vi "Set IPS Switch Heater.vi"(8 "error in (no error)":errorcluster, 10 "Switch Heater Status":T1, 11 "Instrument.Oxford1820 in":refnum<class "Instrument.Oxford1820.lvclass">) -> (0 "error out":errorcluster, 2 "Response":string, 3 "Instrument.Oxford1820 out":refnum<class "Instrument.Oxford1820.lvclass">)   [LabVIEW 2019, in "Instrument.Oxford1820.lvclass"]
uses:
  Instrument.Oxford1820.lvclass
  <instrlib>/Mercury iXX/Mercury iXX.lvlib
  <instrlib>/Mercury iXX/Public/Libraries/Magnet/Open/Open Magnet Device.vi
  <instrlib>/Mercury iXX/Public/Libraries/Magnet.lvlib
  <instrlib>/Mercury iXX/Public/Libraries/Magnet/Signals/Read/Persistant Current (Read).vi
  <instrlib>/Mercury iXX/Public/Libraries/Magnet/Signals/Read/Current (Read).vi
  <instrlib>/Mercury iXX/Public/Libraries/Magnet/Signals/Set/Switch Heater Status (Set).vi
  <instrlib>/Mercury iXX/Public/Controls/Response String.ctl
  <instrlib>/Mercury iXX/Public/Libraries/Magnet/Controls/Switch Heater.ctl
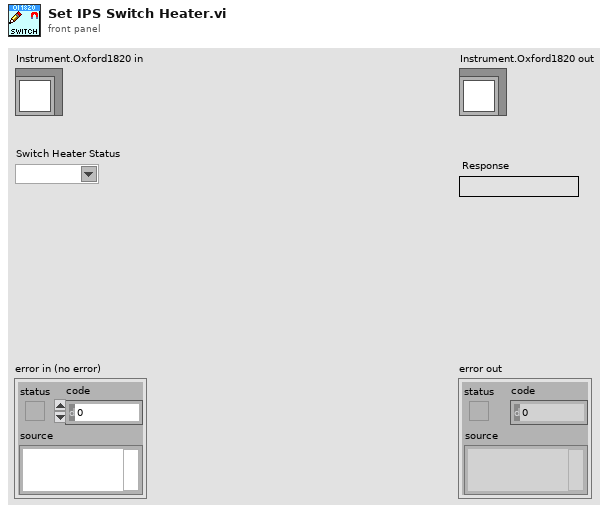
[diagram p1: front panel]
types:
  T1 = typedef "Mercury iXX.lvlib/Magnet.lvlib/Switch Heater.ctl" = string
  T2 = typedef "Mercury iXX.lvlib/Response String.ctl" = string
  T3 = typedef "Mercury iXX.lvlib/Mercury Reference.ctl" = cluster{"Comms":refnum<visa-resource-name>, "Device ID":string[], "Comms Layer":T4, "Command":string, "Query reference":T5}
  T4 = typedef "Mercury iXX.lvlib/Comms Transport Layer.ctl" = enum16{"Ethernet TCP/IP", "USB", "ISOBus - RS-232", "GPIB"}
  T5 = typedef "Mercury iXX.lvlib/Query Dynamic Reference.ctl" = refnum<vi>
  T6 = typedef "Mercury iXX.lvlib/Is Valid LED.ctl" = bool
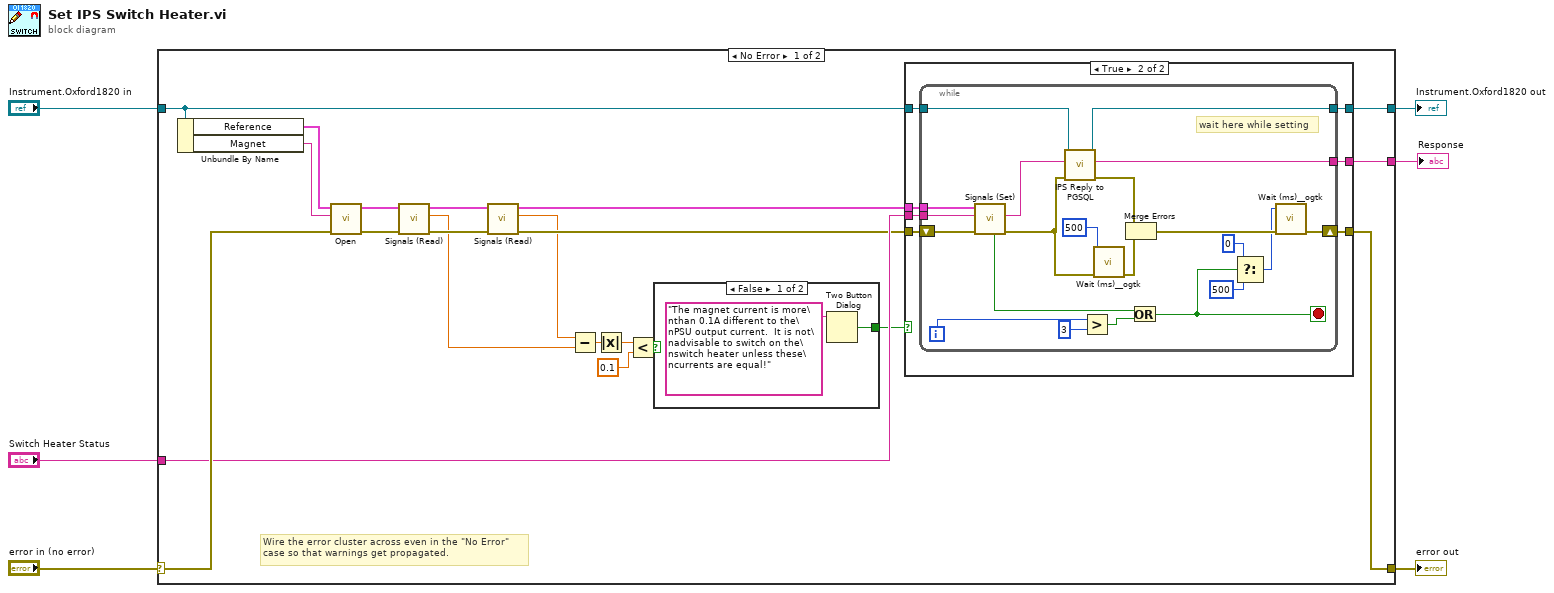
[diagram p0: block diagram]
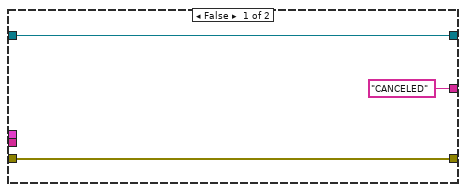
[diagram p2: hidden frame]
diagram:
  n1 = case shown="No Error" "error in (no error)" {
    selector: "error in (no error)" -> [w15 w62]
    tunnel: [w27 w62] -> w5
    tunnel: [w7 w61] -> w3
    tunnel: "Instrument.Oxford1820 in" -> [w8 w61]
    tunnel: [w26 _] -> w2
    tunnel: "Switch Heater Status" -> [w14 _]
    frame No Error {
      # "Wire the error cluster across even in the \"No Error\"\ncase so that warnings get propagated."
      n2 = Unbundle By Name(w8) -> ("Reference"=w25:T3, "Magnet"=w24:string)
      n3 = call-poly <instrlib>:"Open.vi"("error in (no error)"=w15, "Device Identifier"=w24, "Mercury Reference In"=w25) -> ("error out"=w18:errorcluster, "Mercury Reference Out"=w17:T3)  [unwired: 7 out]
      n4 = call-poly <instrlib>:"Signals (Read).vi"("error in"=w18, "Mercury Reference In"=w17) -> ("error out"=w20:errorcluster, "Current"=w10:dbl, "Mercury Reference Out"=w19:T3)  [unwired: 1 in, 6 out]
      n5 = call-poly <instrlib>:"Signals (Read).vi"("error in"=w20, "Mercury Reference In"=w19) -> ("error out"=w13:errorcluster, "Persistant Current"=w11:dbl, "Mercury Reference Out"=w12:T3)  [unwired: 1 in, 6 out]
      n6 = Subtract(x=w11, y=w10) -> (x-y=w21:dbl)
      n7 = Absolute Value(x=w21) -> (abs(x)=w22:dbl)
      n8 = Less?(x=w22, y=0.1) -> (x < y?=w23:bool)
      n9 = case shown="False" w23 {
        selector: w23 -> [_ w60]
        tunnel: [w59 w60] -> w9
        frame False {
          n10 = Two Button Dialog(message="The magnet current is more\nthan 0.1A different to the\nPSU output current.  It is not\nadvisable to switch on the\nswitch heater unless these\ncurrents are equal!") -> (T button?=w59:bool)  [unwired: 2 out]
        }
        frame True {
        }
      }
      n11 = case shown="True" w9 {
        tunnel: [w30 w37] -> w27
        tunnel: [T2 "CANCELED" ("Response") w36] -> w26
        tunnel: w8 -> [w28 w35]
        tunnel: w14 -> [_ w34]
        tunnel: w13 -> [w30 w33]
        tunnel: w12 -> [_ w32]
        tunnel: [w28 w31] -> w7
        frame False {
        }
        frame True {
          n12 = while {
            tunnel: [w46] -> w36
            tunnel: w35 -> [w48]
            tunnel: w34 -> [w55]
            tunnel: w32 -> [w56]
            shift-right: [w53] -> w37
            shift-left: w33 -> [w57]
            tunnel: [w47] -> w31
            i -> [w42]
            stop <- w40 stop-if-true
            # "wait here while setting"
            n13 = call-poly <instrlib>:"Signals (Set).vi"("error in"=w57, "Switch Heater Status"=w55, "Mercury Reference In"=w56) -> ("error out"=w51:errorcluster, "Response"=w46:T2, "Valid?"=w39:T6)  [unwired: 1 in, 5 out]
            n14 = call "IPS Reply to PGSQL.vi"("error in (no error)"=w51, "Response"=w46, "Instrument.1820 in"=w48) -> ("error out"=w50:errorcluster, "Instrument.1820 out"=w47:refnum<class "Instrument.Oxford1820.lvclass">)  [unwired: 7 in]
            n15 = Greater?(x=w42, y=3) -> (0:w38:bool)
            n16 = call <userlib>:"Wait (ms)__ogtk.vi"("error in (no error)"=w51, "milliseconds to wait"=u32 500) -> ("error out"=w49:errorcluster)  [unwired: 8 in, 1 out]
            n17 = Merge Errors(w50, w49) -> (w52:errorcluster)
            n18 = Or(x=w39, y=w38) -> (x .or. y?=w40:T6)
            n19 = Select(t=u32 0, s=w40, f=u32 500 ("milliseconds to wait")) -> (s? t:f=w43:u32)
            n20 = call <userlib>:"Wait (ms)__ogtk.vi"("error in (no error)"=w52, "milliseconds to wait"=w43) -> ("error out"=w53:errorcluster)  [unwired: 8 in, 1 out]
          }
        }
      }
    }
    frame Error {
    }
  }
  "error out" <- w5
  "Instrument.Oxford1820 out" <- w3
  "Response" <- w2
